vi "Run 04.vi"(11 "NXT/EV3 in":T1) -> (3 "EV3 out":T1)   [LabVIEW 2016]
uses:
  <vilib>/NXT/Subs/LVHSConnector.ctl
  <vilib>/NXT/LegoClasses/BrickReference/BrickReference.lvclass
  <vilib>/NXT/Block Support/NXT_ButtonSelector.ctl
  <vilib>/NXT/Dual Mode Library/Waits/Wait_Btn_Press.vi
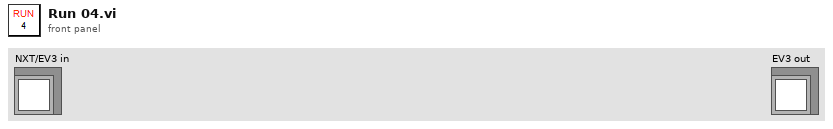
[diagram p1: front panel]
types:
  T1 = typedef "LVHSConnector.ctl" = refnum<class "BrickReference.lvclass">
  T2 = typedef "NXT_ButtonSelector.ctl" = u16
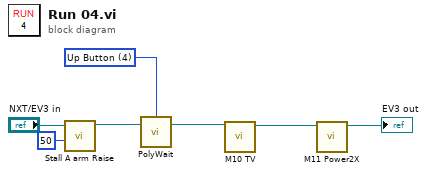
[diagram p0: block diagram]
diagram:
  w1 = T2 4 items=["Enter button"=3, "Left button"=2, "Right button"=1, "Up Button"=4, "Down Button"=5] ("Button (Enter button)")
  n1 = call "Stall A arm Raise.vi"("Power"=i8 50, "NXT/EV3"="NXT/EV3 in") -> ("NXT/EV3"=w5:T1)  [unwired: 9 in]
  n2 = call-poly <vilib>:"PolyWait.vi"("NXT/EV3"=w5, "Button (Enter button)"=w1) -> ("NXT/EV3"=w2:T1)  [unwired: 2 in]
  n3 = call "M10 TV.vi"("NXT/EV3"=w2) -> ("EV3 out"=w7:T1)  [unwired: 10 in]
  n4 = call "M11 Power2X.vi"("NXT/EV3"=w7) -> ("EV3 out"=→"EV3 out":T1)  [unwired: 10 in]
